vi "ResetK2182andK6221.vi"(11 "KEITHLEY 2182 & KEITHLEY 6221_In":refnum<vi>) -> (3 "KEITHLEY 2182 & KEITHLEY 6221_Out":refnum<vi>)   [LabVIEW 2013]
uses:
  Keithley 622x lib/Typedefs/KE622x -- On Off Control.ctl
  Keithley 622x lib/Keithly user program.lvlib
panel:
  out "error out":errorcluster
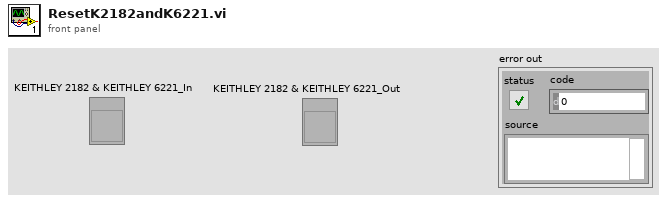
[diagram p1: front panel]
types:
  T1 = typedef "Keithly user program.lvlib/KE622x -- On Off Control.ctl" = enum16{"Off", "On"}
  T2 = typedef "Keithly user program.lvlib/KE2182 -- Params.ctl" = cluster{"Auto Range?":bool, "Man / Selected\n       Range":enum16{"10mV", "100mV", "1V", "10V", "100V"}, "Enable Digital\n       Filter?":bool, "Filter Type":enum16{"Movin", "Repeat"}, "Filter Count":u32, "      Filter\nWindow (%)":dbl, "Enable Analog\n       Filter?":bool, "NPLCs":u32}
  T3 = typedef "Keithly user program.lvlib/KE622x -- Current Range.ctl" = cluster{"Auto Range?":bool, "Man / Selected\n        Range":enum16{"2nA", "20nA", "200nA", "2uA", "20uA", "200uA", "2mA", "20mA", "100mA"}}
  T4 = typedef "Keithly user program.lvlib/KE622x -- Current Level.ctl" = dbl
  T5 = typedef "Keithly user program.lvlib/KE622x -- Voltage Limit.ctl" = dbl
  T6 = typedef "Keithly user program.lvlib/KE6221 -- Output Response.ctl" = enum16{"Fast", "Slow"}
  T7 = cluster{"KEITHLEY ON/OFF":bool, "VISA KEITHLEY resource name":refnum<visa-resource-name>, "2182 -A Params":T2, "KEITHLEY CURRENT ON/OFF":bool, "6221 Params":cluster{"Current Range":T3, "Current Level (A)":T4, "Voltage Limit (V)":T5, "KE6221 Output Response":T6, "Analog Filter State":enum16{"Off", "On"}}, "Step Mode\nParams":bool, "Step Mode":cluster{"Front Point (A)":T4, "Start Point (A)":T4, "Back Point (A)":T4, "Step(A)":T4, "Time step (ms)":dbl, "N cycle":i32, "Sweeping":enum16{"Off Sweeping", "On Sweeping"}, "Go to":enum16{"Star Point", "Back Point"}}}
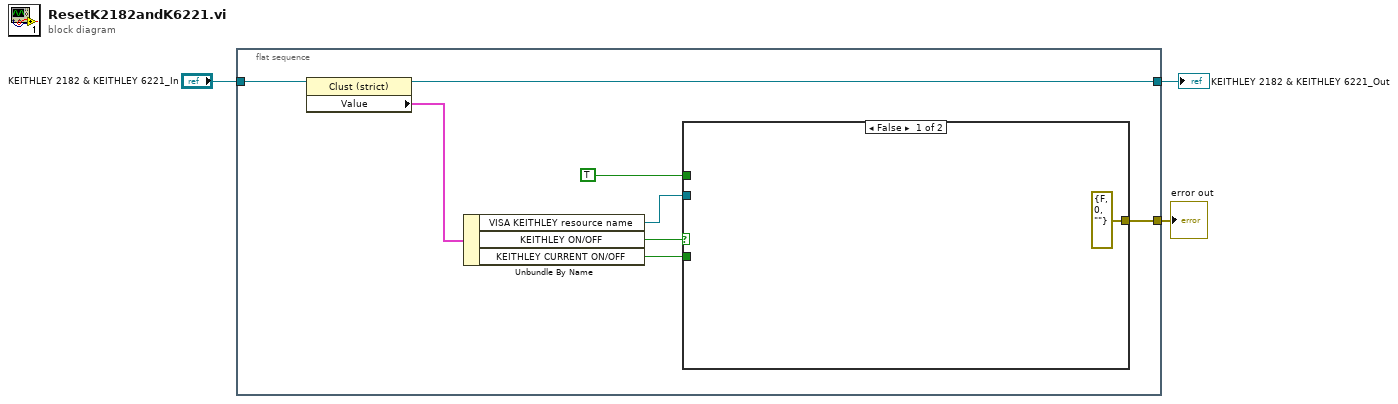
[diagram p0: block diagram]
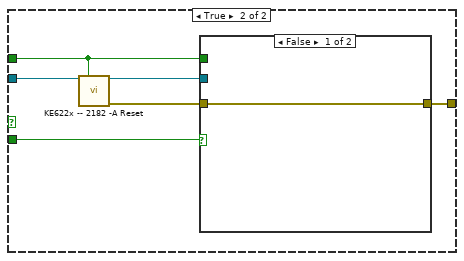
[diagram p2: hidden frame]
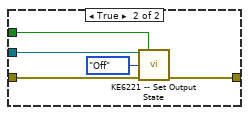
[diagram p3: hidden frame]
diagram:
  n1 = flat-sequence {
    tunnel: "KEITHLEY 2182 & KEITHLEY 6221_In" -> [w11]
    tunnel: [w10] -> w3
    tunnel: [w4] -> w1
    frame #0 {
      n2 = property class="Clust (strict)"(reference=w11) -> (reference out=w10:refnum<vi>, "Value"=w9:T7)  [unwired: 1 in, 1 out]
      n3 = Unbundle By Name(w9) -> ("VISA KEITHLEY resource name"=w7:refnum<visa-resource-name>, "KEITHLEY ON/OFF"=w8:bool, "KEITHLEY CURRENT ON/OFF"=w5:bool)
      n4 = case shown="False" w8 {
        tunnel: w7 -> [_ w18]
        tunnel: TRUE -> [_ w14]
        tunnel: w5 -> [_ w17]
        tunnel: [errorcluster {"status"=FALSE, "code"=0, "source"=""} ("error out") w13] -> w4
        frame False {
        }
        frame True {
          n5 = call "KE622x -- 2182 -A Reset.vi"("622x Resource In"=w18, "Check For SCPI Errors? (T)"=w14) -> ("622x Resource Out (dupl)"=w16:refnum<visa-resource-name>, "error out"=w15:errorcluster)  [unwired: 12 in]
          n6 = case shown="False" w17 {
            tunnel: w16 -> [_ w24]
            tunnel: w15 -> [w19 w23]
            tunnel: w14 -> [_ w21]
            tunnel: [w19 w20] -> w13
            frame False {
            }
            frame True {
              n7 = call "KE6221 -- Set Output State.vi"("Resource In"=w24, "Check For SCPI Errors? (T)"=w21, "Output State"=KE622x_--_On_Off_Control."Off", "error in (no error)"=w23) -> ("error out"=w20:errorcluster)  [unwired: 10 in, 1 out]
            }
          }
        }
      }
    }
  }
  "KEITHLEY 2182 & KEITHLEY 6221_Out" <- w3
  "error out" <- w1
